vi "ProgramControl.vi"(0 "Universal Robot.lvclass in":refnum<class "Universal Robot.lvclass">, 1 "Program":string, 5 "error in (no error)":errorcluster, 8 "Timeout (s)":dbl=-1.0, 9 "Subpanel":refnum<vi>, 11 "Require Normal Mode to Play (F)":bool) -> (14 "Universal Robot.lvclass out":refnum<class "Universal Robot.lvclass">, 15 "programReturnStatus":T1=enum."Complete", 19 "error out":errorcluster)   [LabVIEW 2019, in "Universal Robot.lvclass"]
uses:
  Universal Robot.lvclass
  ProgramReturnStatus.ctl
  ProgramControlFPControls.ctl
  ProgramState.ctl
  Events/Robot Event/Event Type.ctl
  ProgramControlEvent.ctl
  Events/Robot Event/Robot Event.lvclass
panel:
  out "Loaded Program":string
  out "Program Status":string
  out "Program Status Color":u32(colorbox)
  out "Safety Status":string
  out "Safety Status Color":u32(colorbox)
  out "Time Elapsed":string
  out "Message":string
  in  "Abort":bool
  in  "Resume":bool
  in  "check status timeout":i32=1000
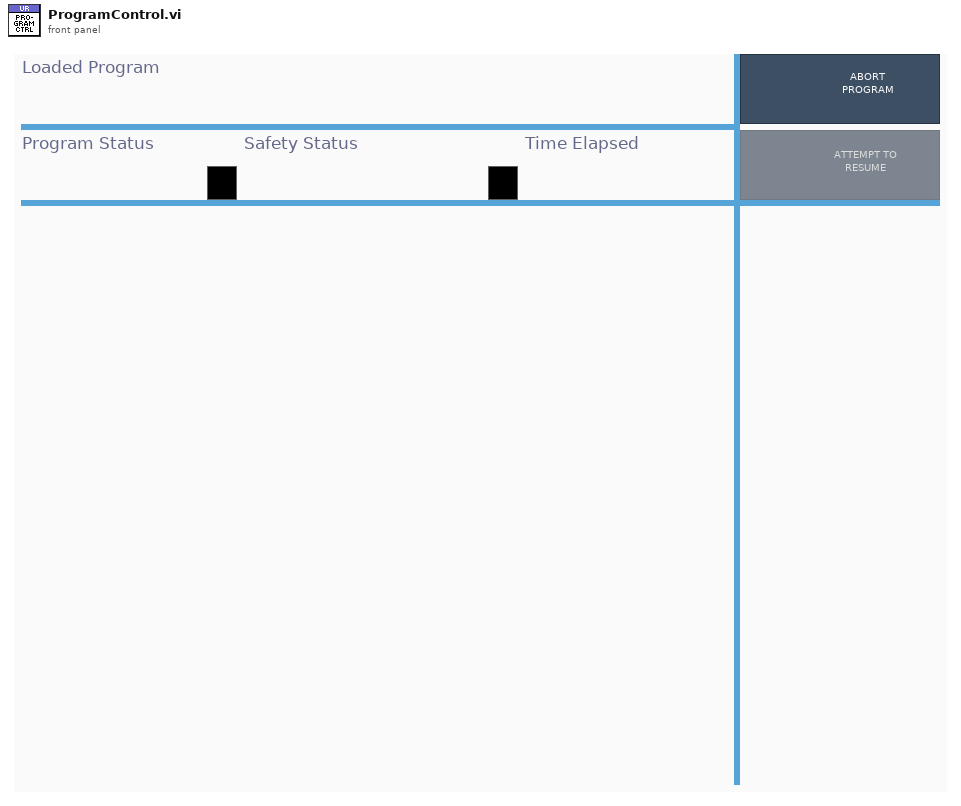
[diagram p1: front panel]
types:
  T1 = typedef "Universal Robot.lvclass/ProgramReturnStatus.ctl" = enum16{"Incomplete", "Complete", "Stopped", "User Stopped", "Error", "Faulted", "Timeout"}
  T2 = typedef "Universal Robot.lvclass/ProgramControlFPControls.ctl" = cluster{"Recover Button":refnum<vi>, "Resume Bottom":refnum<vi>, "Message":refnum<vi>, "Program Status":refnum<vi>, "Loaded Program":refnum<vi>, "VI Reference":refnum<vi>, "Time Elapsed":refnum<vi>, "Safety Status":refnum<vi>, "Program Status Color":refnum<vi>, "Safety Status Color":refnum<vi>}
  T3 = typedef "Universal Robot.lvclass/ProgramState.ctl" = enum16{"STOPPED", "PLAYING", "PAUSE"}
  T4 = typedef "Robot Event.lvclass/Event Type.ctl" = enum16{"Play", "Error", "Fault", "Timeout", "Stopped", "Complete", "Fault - Program Resumed", "Fault - Program Aborted"}
  T5 = typedef "Universal Robot.lvclass/ProgramControlEvent.ctl" = enum16{"Stop", "Pause", "Resume"}
  T6 = typedef "Universal Robot.lvclass/ProgramStatus.ctl" = cluster{"Loaded Program":string, "Valid Program":bool, "Program State":T3, "Running":bool}
  T7 = typedef "Universal Robot.lvclass/SafetyStatus.ctl" = enum16{"INVALID", "NORMAL", "REDUCED", "PROTECTIVE_STOP", "RECOVERY", "SAFEGUARD_STOP", "SYSTEM_EMERGENCY_STOP", "ROBOT_EMERGENCY_STOP", "VIOLATION", "FAULT", "AUTOMATIC_MODE_SAFEGAURD_STOP", "SYSTEM_THREE_POSITION_ENABLING_STOP"}
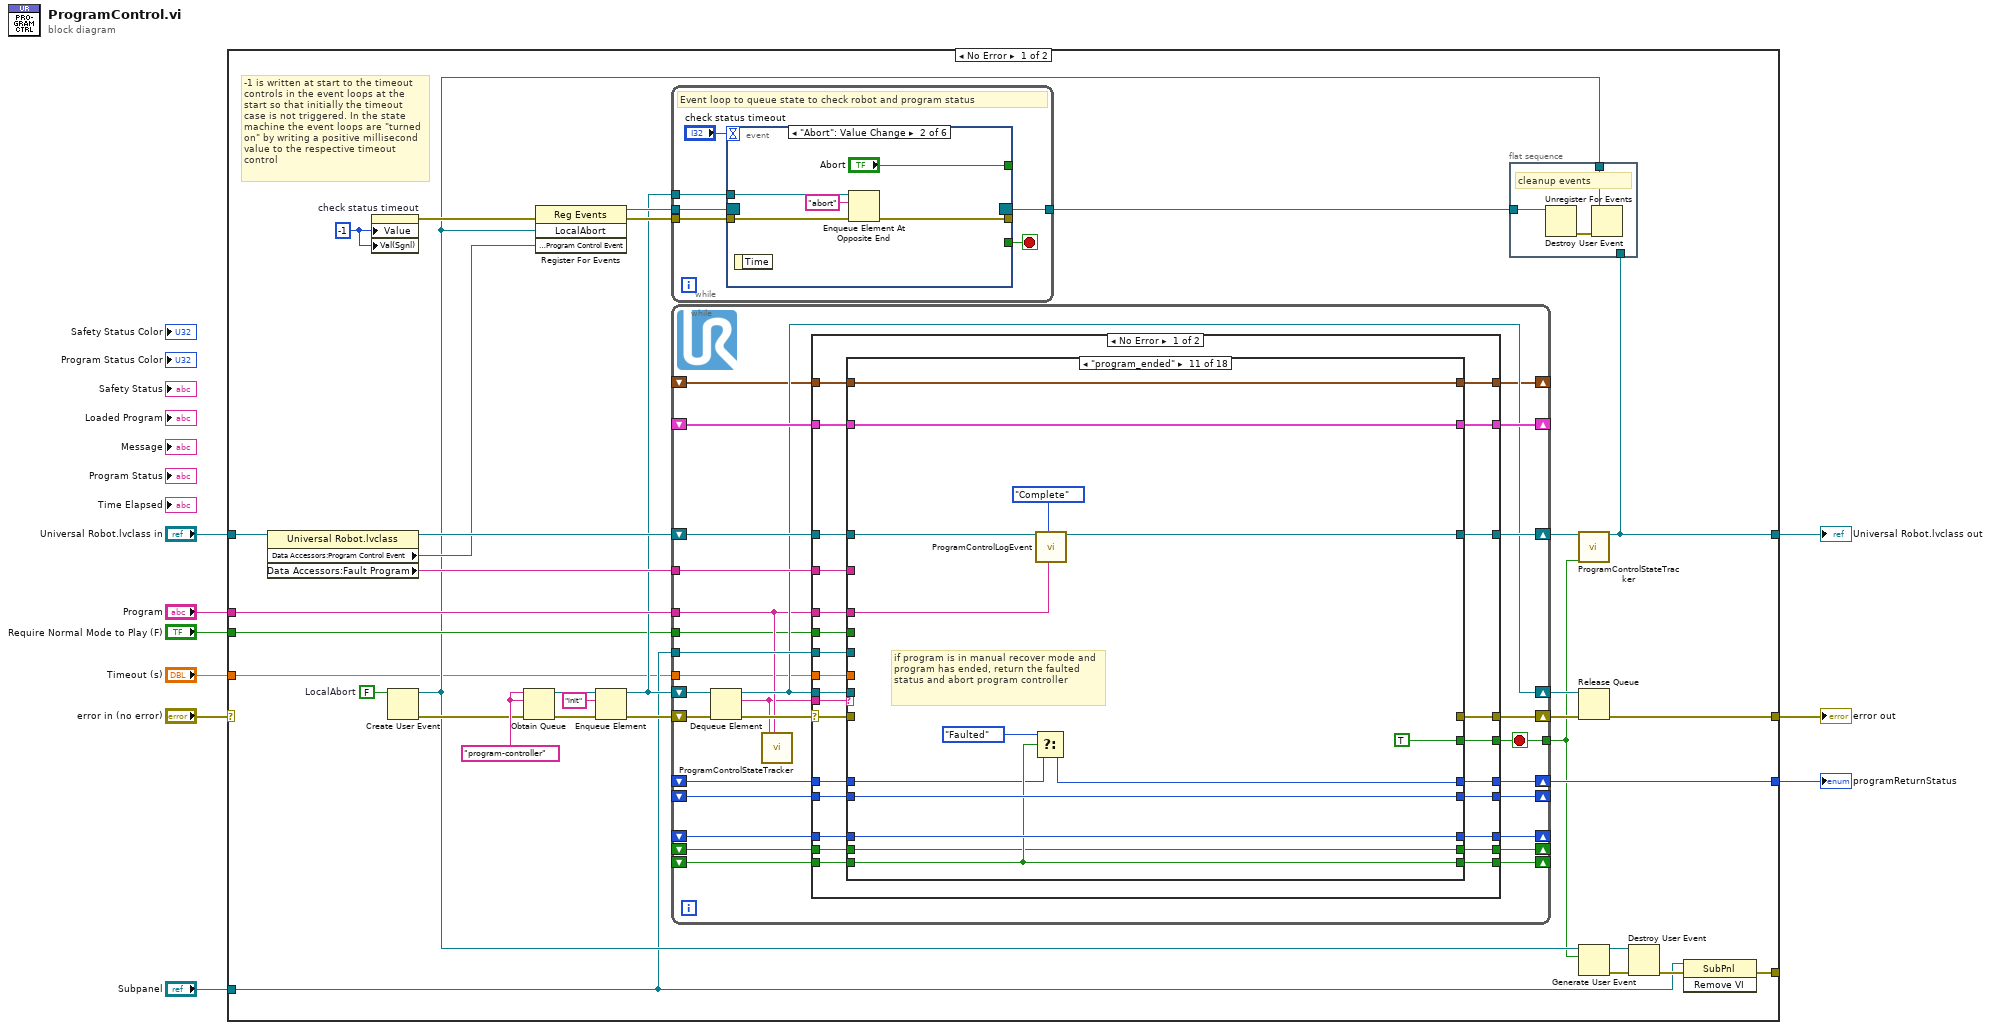
[diagram p0: block diagram]
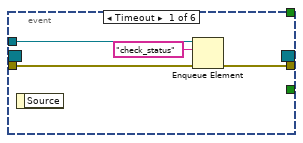
[diagram p2: hidden frame]
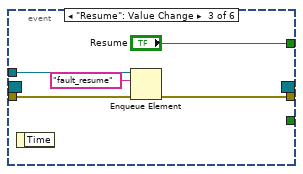
[diagram p3: hidden frame]
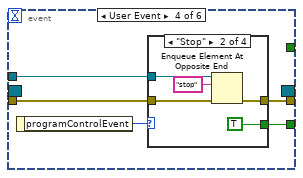
[diagram p4: hidden frame]
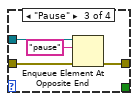
[diagram p6: hidden frame]
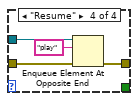
[diagram p7: hidden frame]
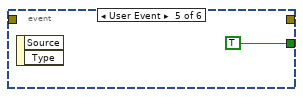
[diagram p8: hidden frame]
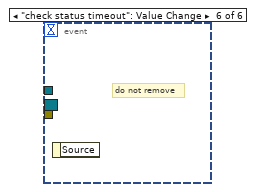
[diagram p9: hidden frame]
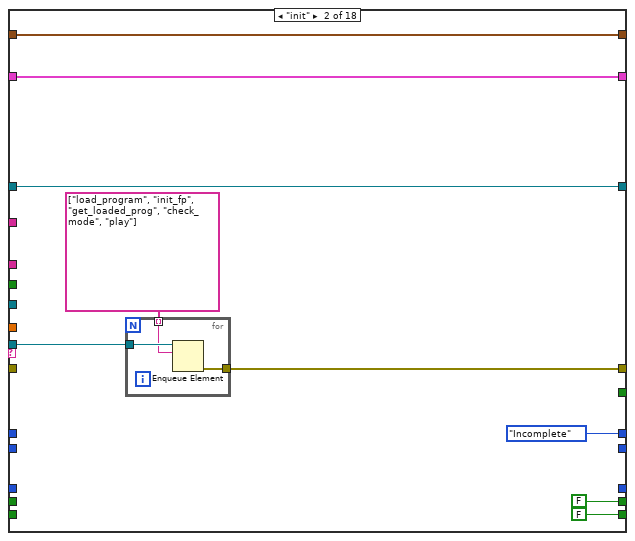
[diagram p11: hidden frame]
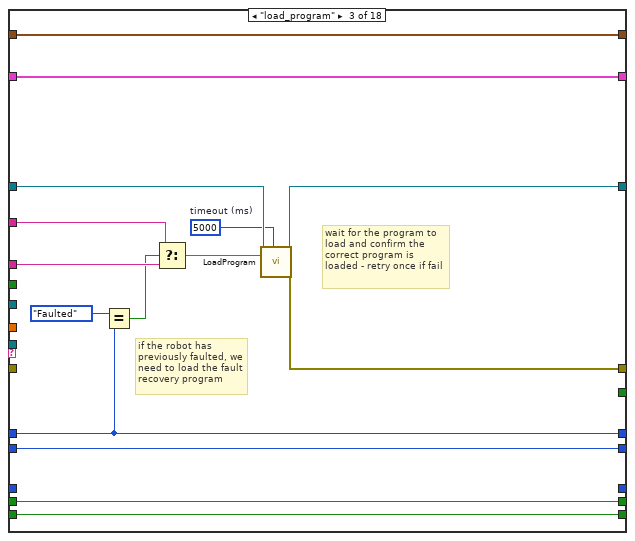
[diagram p12: hidden frame]
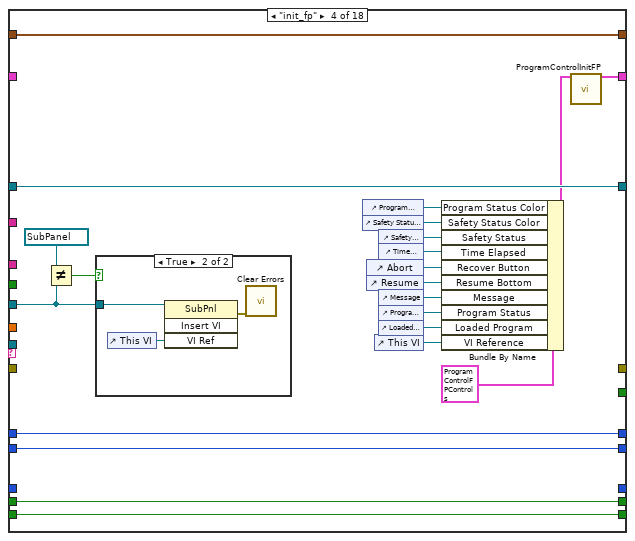
[diagram p13: hidden frame]
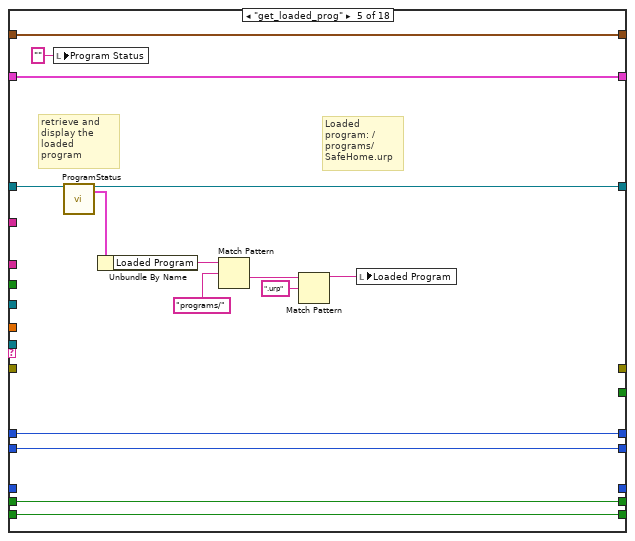
[diagram p15: hidden frame]
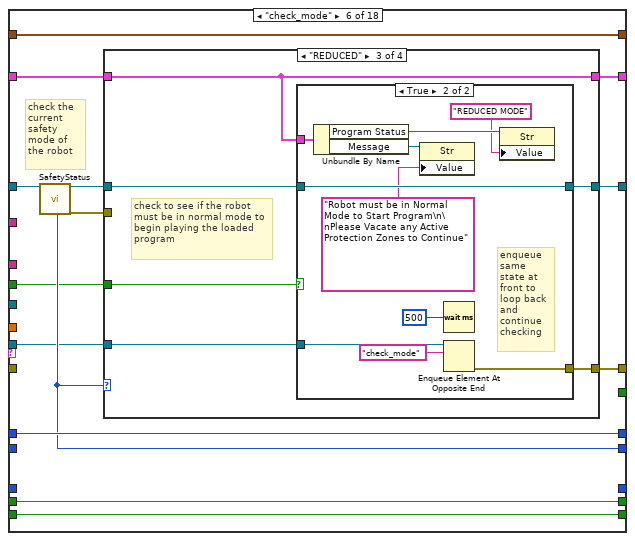
[diagram p16: hidden frame]
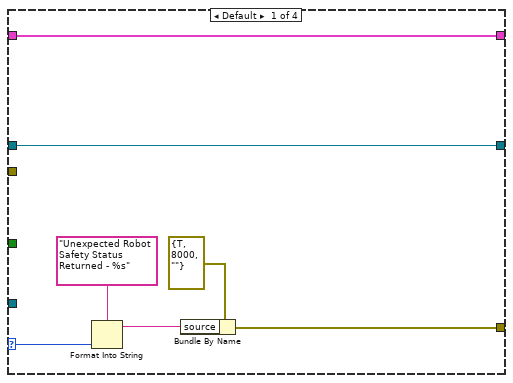
[diagram p17: hidden frame]
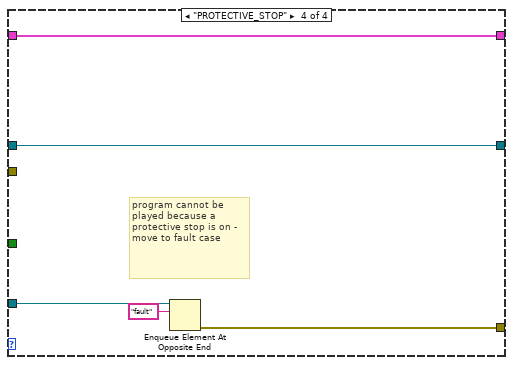
[diagram p20: hidden frame]
diagram:
  n1 = case shown="No Error" "error in (no error)" {
    selector: "error in (no error)" -> [_ w564]
    tunnel: "Universal Robot.lvclass in" -> [w33 w563]
    tunnel: [w31 _] -> w8
    tunnel: [w24 w564] -> w7
    tunnel: [w15 w563] -> w6
    tunnel: "Subpanel" -> [w12 _]
    tunnel: "Program" -> [w23 _]
    tunnel: "Require Normal Mode to Play (F)" -> [w18 _]
    tunnel: [w11 _] -> _
    tunnel: "Timeout (s)" -> [w10 _]
    frame No Error {
      w30 = FALSE  # LocalAbort
      w20 = -1 ("rate")
      w38 = "program-controller" ("name (unnamed)")
      # "-1 is written at start to the timeout controls in the event loops at the start so that initially the timeout case is not triggered. In the state machine the event loops are \"turned on\" by writing a positive millisecond value to the respective timeout control"
      n2 = property class="Universal Robot.lvclass"(reference=w33) -> (reference out=w37:refnum<class "Universal Robot.lvclass">, "Data Accessors:Program Control Event"=w32:refnum<user-event>, "Data Accessors:Fault Program"=w22:string)  [unwired: 1 in, 1 out]
      n3 = property on="check status timeout" class="DigNum (strict)"("Value"=w20, "Val(Sgnl)"=w20) -> (error out=w29:errorcluster)  [unwired: 2 in, 1 out]
      n4 = Create User Event(user event datatype=w30) -> (user event=w16:refnum<user-event>, error out=w28:errorcluster)  [unwired: 1 in]
      n5 = Obtain Queue(name (unnamed)=w38, element data type=w38, error in (no error)=w28) -> (queue out=w36:refnum<queue>, error out=w35:errorcluster)  [unwired: 2 in, 1 out]
      n6 = register-events(error in=w29, w16, w32) -> (reference out=w42:refnum<event-registration>, error out=w41:errorcluster)  [unwired: 1 in]
      n7 = Enqueue Element(queue=w36, element="init", error in (no error)=w35) -> (queue out=w21:refnum<queue>, error out=w34:errorcluster)  [unwired: 1 in, 1 out]
      n8 = while {
        tunnel: w21 -> [w51]
        tunnel: w41 -> [w50]
        tunnel: w42 -> [w49]
        tunnel: [w47] -> w17
        stop <- w46 stop-if-true
        # "Event loop to queue state to check robot and program status"
        n9 = event shown="[1] \"Abort\": Value Change" {
          selector: w49 -> [_ _ _ _ _ _]
          dyn-events: [_ _ _ _ _ _] -> w47
          timeout: "check status timeout" -> [_ _ _ _ _ _]
          tunnel: w51 -> [w55 w60 w65 w70 _ _]
          tunnel: w50 -> [w54 w59 w64 w69 _ _]
          tunnel: [w53 w58 w63 w68 _ _] -> _
          tunnel: [_ _ _ w66 TRUE _] -> w46
          tunnel: [_ "Abort" "Resume" _ _ _] -> _
          event Timeout {
            n10 = event-data() -> ()  [unwired: 1 in, 1 out]
            n11 = Enqueue Element(queue=w55, element="check_status", error in (no error)=w54) -> (error out=w53:errorcluster)  [unwired: 1 in, 2 out]
          }
          event "Abort": Value Change {
            n12 = event-data() -> ()  [unwired: 1 in, 1 out]
            n13 = Enqueue Element At Opposite End(queue=w60, element="abort", error in (no error)=w59) -> (error out=w58:errorcluster)  [unwired: 1 in, 2 out]
          }
          event "Resume": Value Change {
            n14 = event-data() -> ()  [unwired: 1 in, 1 out]
            n15 = Enqueue Element(queue=w65, element="fault_resume", error in (no error)=w64) -> (error out=w63:errorcluster)  [unwired: 1 in, 2 out]
          }
          event User Event {
            n16 = event-data() -> ("programControlEvent"=w67:T5)  [unwired: 1 in]
            n17 = case shown="\"Stop\"" w67 {
              tunnel: w70 -> [_ w76 w80 w84]
              tunnel: w69 -> [w71 w75 w79 w83]
              tunnel: [w71 w74 w78 w82] -> w68
              tunnel: [_ TRUE _ _] -> w66
              frame Default {
              }
              frame "Stop" {
                n18 = Enqueue Element At Opposite End(queue=w76, element="stop", error in (no error)=w75) -> (error out=w74:errorcluster)  [unwired: 1 in, 2 out]
              }
              frame "Pause" {
                n19 = Enqueue Element At Opposite End(queue=w80, element="pause", error in (no error)=w79) -> (error out=w78:errorcluster)  [unwired: 1 in, 2 out]
              }
              frame "Resume" {
                n20 = Enqueue Element At Opposite End(queue=w84, element="play", error in (no error)=w83) -> (error out=w82:errorcluster)  [unwired: 1 in, 2 out]
              }
            }
          }
          event User Event {
            n21 = event-data() -> ()  [unwired: 1 in, 2 out]
          }
          event "check status timeout": Value Change {
            # "do not remove"
            n22 = event-data() -> ()  [unwired: 1 in, 1 out]
          }
        }
      }
      n23 = while {
        shift-right: [w113] -> w40
        shift-left: w34 -> [w100]
        shift-right: [w99] -> w39
        shift-left: w21 -> [w101]
        shift-right: [w111] -> w19
        shift-left: w37 -> [w112]
        tunnel: [w109] -> w14
        tunnel: w12 -> [w108]
        shift-right: [w107] -> _
        shift-left: _ -> [w106]
        tunnel: w23 -> [w97]
        tunnel: w22 -> [w105]
        shift-right: [w110] -> w31
        shift-left: _ -> [w104]
        shift-right: [w103] -> _
        shift-left: _ -> [w102]
        tunnel: w18 -> [w96]
        shift-right: [w94] -> _
        shift-left: _ -> [w93]
        shift-right: [w92] -> _
        shift-left: _ -> [w91]
        tunnel: w10 -> [w90]
        shift-right: [w89] -> _
        shift-left: _ -> [w88]
        shift-right: [w87] -> _
        shift-left: _ -> [w86]
        stop <- w109 stop-if-true
        n24 = Dequeue Element(queue=w101, error in (no error)=w100) -> (queue out=w99:refnum<queue>, element=w95:string, error out=w98:errorcluster)  [unwired: 1 in, 1 out]
        n25 = call "ProgramControlStateTracker.vi"("State in"=w95, "Program"=w97) -> ()  [unwired: 17 in, 1 out]
        n26 = case shown="No Error" w98 {
          selector: w98 -> [w125 w557]
          tunnel: w99 -> [w126 _]
          tunnel: [w139 w557] -> w113
          tunnel: [w138 TRUE] -> w109
          tunnel: w112 -> [w137 w554]
          tunnel: [w136 w552] -> w111
          tunnel: [w135 ProgramReturnStatus."Error" ("programReturnStatus")] -> w110
          tunnel: w108 -> [w134 _]
          tunnel: [w133 w560] -> w107
          tunnel: w106 -> [w132 w560]
          tunnel: w97 -> [w129 w551]
          tunnel: w105 -> [w131 _]
          tunnel: w104 -> [w130 _]
          tunnel: [w128 w559] -> w103
          tunnel: w102 -> [w127 w559]
          tunnel: w95 -> [w124 _]
          tunnel: w96 -> [w123 _]
          tunnel: [w122 w549] -> w94
          tunnel: w93 -> [w121 w549]
          tunnel: [w120 w550] -> w92
          tunnel: w91 -> [w119 w550]
          tunnel: w90 -> [w118 _]
          tunnel: [w117 w548] -> w89
          tunnel: w88 -> [w116 w548]
          tunnel: [w115 w547] -> w87
          tunnel: w86 -> [w114 w547]
          frame No Error {
            n27 = case shown="\"program_ended\"" w124 {
              tunnel: w125 -> [w147 _ _ _ _ _ _ _ _ _ _ w405 w428 _ w459 _ _ _]
              tunnel: w126 -> [_ w154 _ _ _ w225 w275 _ _ w331 _ w412 w434 w444 w475 w492 _ _]
              tunnel: [w147 w153 w160 _ _ w226 w276 errorcluster {"status"=TRUE, "code"=8000, "source"="Timed out waiting for program to play"} ("error out") _ w330 _ w401 w418 w443 w464 w487 w531 w542] -> w139
              tunnel: [_ _ _ _ _ _ _ TRUE _ _ TRUE _ _ _ _ w480 TRUE _] -> w138
              tunnel: w137 -> [w146 w156 w173 w187 w214 w223 w280 w302 w310 w323 w387 w410 w433 w442 w468 w489 w532 w546]
              tunnel: [w146 w156 w161 w187 w213 w221 w268 w302 w310 w329 w385 w409 w432 w441 w466 w491 w517 w543] -> w136
              tunnel: [w144 ProgramReturnStatus."Incomplete" ("programReturnStatus") w169 w188 w206 w228 w270 ProgramReturnStatus."Error" ("programReturnStatus") w307 w325 w390 w411 ProgramReturnStatus."Timeout" ("programReturnStatus") w437 w471 ProgramReturnStatus."Faulted" ("programReturnStatus") w520 w538] -> w135
              tunnel: w134 -> [_ _ _ w196 _ _ _ _ _ _ _ _ _ _ _ _ _ _]
              tunnel: [w145 w155 w174 w189 w205 w218 w263 w299 w308 w328 w397 w413 w423 w447 w472 w494 w528 w540] -> w133
              tunnel: w132 -> [w145 w155 w174 _ w205 w219 w263 w299 w308 w320 w397 w414 w423 w447 w473 w494 w528 w540]
              tunnel: w129 -> [_ _ w172 _ _ _ w266 _ _ _ w386 w408 w431 _ w465 w488 w515 _]
              tunnel: w131 -> [_ _ w171 _ _ _ _ _ _ _ _ _ _ _ _ w483 _ _]
              tunnel: w130 -> [w144 _ w169 w188 w206 w228 w270 _ w307 w326 w392 w411 _ w439 w471 _ w521 w538]
              tunnel: [w143 _ w166 w184 w204 w227 w265 w297 w306 w327 w395 w406 w429 w436 w470 w490 w527 w537] -> w128
              tunnel: w127 -> [w143 _ w166 w184 w204 _ w265 w297 w306 w324 w395 w406 w429 w438 w470 w490 w527 w537]
              tunnel: w123 -> [_ _ _ _ _ w220 _ _ _ _ _ _ _ _ _ _ _ _]
              tunnel: [_ _ _ _ _ _ _ _ _ w319 w394 w403 w426 _ _ _ _ _] -> w122
              tunnel: w121 -> [_ _ _ _ _ _ _ _ _ _ w394 w403 w426 _ _ _ _ _]
              tunnel: [w142 FALSE w165 w181 w202 w217 w262 w296 w305 w318 w393 w400 w425 w446 w462 TRUE w526 w536] -> w120
              tunnel: w119 -> [w142 _ w165 w181 w202 w217 w262 w296 w305 w318 w393 w400 w425 w446 w462 w482 w526 w536]
              tunnel: w118 -> [_ _ _ _ _ _ _ _ _ w317 _ _ w422 _ _ _ _ _]
              tunnel: [w141 w149 w164 w180 w201 w216 w261 w295 w304 w315 w389 w399 w424 w445 w461 w486 w525 w535] -> w117
              tunnel: w116 -> [w141 w149 w164 w180 w201 w216 w261 w295 _ w315 w389 w399 w424 w445 w461 w486 w525 w535]
              tunnel: [w140 FALSE w163 w175 w200 w215 FALSE w294 w303 w311 w388 TRUE w416 w440 w460 w479 w519 w534] -> w115
              tunnel: w114 -> [w140 _ w163 w175 w200 w215 _ w294 w303 w311 w388 _ w416 w440 w460 w479 w519 w534]
              frame Default {
              }
              frame "init" {
                n28 = for {
                  tunnel: w154 -> [w159]
                  tunnel: [w158] -> w153
                  tunnel: string[] ["load_program", "init_fp", "get_loaded_prog", "check_mode", "play"] -> [w157] mode=indexing
                  n29 = Enqueue Element(queue=w159, element=w157) -> (error out=w158:errorcluster)  [unwired: 2 in, 2 out]
                }
              }
              frame "load_program" {
                w162 = u32 5000  # timeout (ms)
                # "wait for the program to load and confirm the correct program is loaded - retry once if fail"
                # "if the robot has previously faulted, we need to load the fault recovery program"
                n30 = Equal?(x=ProgramReturnStatus."Faulted", y=w169) -> (x = y?=w167:bool)
                n31 = Select(t=w171, s=w167, f=w172) -> (s? t:f=w170:string)
                n32 = call-dynamic "LoadProgram.vi"("Universal Robot.lvclass in"=w173, "program in"=w170, "timeout (ms)"=w162) -> ("Universal Robot.lvclass out"=w161:refnum<class "Universal Robot.lvclass">, "error out"=w160:errorcluster)  [unwired: 14 in, 1 out]
              }
              frame "init_fp" {
                n33 = Not Equal?(x=refnum<vi> refnum, y=w196) -> (x != y?=w194:bool)
                n34 = case shown="True" w194 {
                  tunnel: w196 -> [_ w199]
                  frame False {
                  }
                  frame True {
                    n35 = control-ref of="This VI"() -> (w197:refnum<vi>)
                    n36 = invoke class="SubPnl" method="Insert VI"(reference=w199, "VI Ref"=w197) -> (error out=w198:errorcluster)  [unwired: 2 in, 3 out]
                    n37 = call <vilib>:"Clear Errors.vi"("error in (no error)"=w198) -> ()  [unwired: 5 in, 2 out]
                  }
                }
                n38 = control-ref of="Program Status Color"() -> (w177:refnum<vi>)
                n39 = control-ref of="Safety Status Color"() -> (w176:refnum<vi>)
                n40 = control-ref of="Abort"() -> (w193:refnum<vi>)
                n41 = control-ref of="Resume"() -> (w192:refnum<vi>)
                n42 = control-ref of="This VI"() -> (w182:refnum<vi>)
                n43 = control-ref of="Safety Status"() -> (w178:refnum<vi>)
                n44 = control-ref of="Time Elapsed"() -> (w179:refnum<vi>)
                n45 = control-ref of="Message"() -> (w191:refnum<vi>)
                n46 = control-ref of="Program Status"() -> (w190:refnum<vi>)
                n47 = control-ref of="Loaded Program"() -> (w183:refnum<vi>)
                n48 = Bundle By Name(cluster=T2 {"Recover Button"=refnum, "Resume Bottom"=refnum, "Message"=refnum, "Program Status"=refnum, "Loaded Program"=refnum, "VI Reference"=refnum, "Time Elapsed"=refnum, "Safety Status"=refnum, "Program Status Color"=refnum, "Safety Status Color"=refnum} ("Front Panel Controls"), "Program Status Color"=w177, "Safety Status Color"=w176, "Safety Status"=w178, "Time Elapsed"=w179, "Recover Button"=w193, "Resume Bottom"=w192, "Message"=w191, "Program Status"=w190, "Loaded Program"=w183, "VI Reference"=w182) -> (w185:T2)
                n49 = call "ProgramControlInitFP.vi"("Front Panel Controls in"=w185) -> ("Front Panel Controls out"=w189:T2)  [unwired: 18 in]
              }
              frame "get_loaded_prog" {
                # "Loaded program: /programs/SafeHome.urp"
                # "retrieve and display the loaded program"
                n50 = local write "Program Status"("" ("Program Status")) -> ()
                n51 = call-dynamic "ProgramStatus.vi"("Universal Robot.lvclass in"=w214) -> ("Universal Robot.lvclass out"=w213:refnum<class "Universal Robot.lvclass">, "Program Status"=w212:T6)  [unwired: 16 in, 1 out]
                n52 = Unbundle By Name(w212) -> ("Loaded Program"=w210:string)
                n53 = Match Pattern(string=w210, regular expression="programs/") -> (after substring=w208:string)  [unwired: 1 in, 3 out]
                n54 = Match Pattern(string=w208, regular expression=".urp") -> (before substring=w203:string)  [unwired: 1 in, 3 out]
                n55 = local write "Loaded Program"(w203) -> ()
              }
              frame "check_mode" {
                # "check the current safety mode of the robot"
                n56 = call-dynamic "SafetyStatus.vi"("Universal Robot.lvclass in"=w223) -> ("safetyStatus out"=w227:T7, "Universal Robot.lvclass out"=w222:refnum<class "Universal Robot.lvclass">, "error out"=w224:errorcluster)  [unwired: 16 in]
                n57 = case shown="\"REDUCED\"" w227 {
                  selector: w227 -> [w231 _ _ _]
                  tunnel: w224 -> [_ _ _ _]
                  tunnel: [w232 _ w242 w258] -> w226
                  tunnel: w225 -> [_ _ w243 w259]
                  tunnel: w222 -> [w230 w237 w240 w256]
                  tunnel: [w230 w237 w241 w256] -> w221
                  tunnel: w220 -> [_ _ w239 _]
                  tunnel: w219 -> [w229 w236 w238 w255]
                  tunnel: [w229 w236 w238 w255] -> w218
                  frame Default {
                    n58 = Format Into String(format string="Unexpected Robot Safety Status Returned - %s", w231) -> (resulting string=w235:string)  [unwired: 2 in, 1 out]
                    n59 = Bundle By Name(cluster=errorcluster {"status"=TRUE, "code"=8000, "source"=""} ("error constant"), "source"=w235) -> (w232:errorcluster)
                  }
                  frame "NORMAL" {
                  }
                  frame "REDUCED" {
                    # "check to see if the robot must be in normal mode to begin playing the loaded program"
                    n60 = case shown="True" w239 {
                      tunnel: w243 -> [_ w254]
                      tunnel: [_ w253] -> w242
                      tunnel: w240 -> [w244 w249]
                      tunnel: [w244 w249] -> w241
                      tunnel: w238 -> [_ w247]
                      frame False {
                      }
                      frame True {
                        # "enqueue same state at front to loop back and continue checking"
                        n61 = Unbundle By Name(w247) -> ("Program Status"=w246:refnum<vi>, "Message"=w250:refnum<vi>)
                        n62 = property class="Str"(reference=w250, "Value"="Robot must be in Normal Mode to Start Program\n\nPlease Vacate any Active Protection Zones to Continue" ("element")) -> ()  [unwired: 1 in, 2 out]
                        n63 = Wait (ms)(milliseconds to wait=u32 500) -> ()  [unwired: 1 out]
                        n64 = Enqueue Element At Opposite End(queue=w254, element="check_mode") -> (error out=w253:errorcluster)  [unwired: 2 in, 2 out]
                        n65 = property class="Str"(reference=w246, "Value"="REDUCED MODE" ("element")) -> ()  [unwired: 1 in, 2 out]
                      }
                    }
                  }
                  frame "PROTECTIVE_STOP" {
                    # "program cannot be played because a protective stop is on - move to fault case"
                    n66 = Enqueue Element At Opposite End(queue=w259, element="fault") -> (error out=w258:errorcluster)  [unwired: 2 in, 2 out]
                  }
                }
              }
              frame "play" {
                # "play the program and wait  until it begins playing or a timeout is reached"
                n67 = call-dynamic "Play.vi"("Universal Robot.lvclass in"=w280) -> ("Universal Robot.lvclass out"=w279:refnum<class "Universal Robot.lvclass">, "error out"=w278:errorcluster)  [unwired: 17 in]
                n68 = Tick Count (ms)() -> (millisecond timer value=w277:u32)
                n69 = while {
                  shift-right: [w282] -> w269
                  shift-left: w279 -> [w285]
                  tunnel: w278 -> [w284]
                  tunnel: w277 -> [w292]
                  tunnel: [w283] -> w264
                  tunnel: [w290] -> w274
                  tunnel: [w286] -> w267
                  stop <- w287 stop-if-true
                  # "Wait for program to start"
                  n70 = call-dynamic "ProgramState.vi"("Universal Robot.lvclass in"=w285, "error in (no error)"=w284) -> ("Universal Robot.lvclass out"=w282:refnum<class "Universal Robot.lvclass">, "programState out"=w281:T3, "error out"=w283:errorcluster)  [unwired: 15 in]
                  n71 = Tick Count (ms)() -> (millisecond timer value=w293:u32)
                  n72 = Subtract(x=w293, y=w292) -> (x-y=w286:u32)
                  n73 = Greater?(x=w286, y=u32 5000) -> (0:w290:bool)
                  n74 = Equal?(x=ProgramState."PLAYING", y=w281) -> (x = y?=w288:bool)
                  n75 = Or(x=w288, y=w290) -> (x .or. y?=w287:bool)
                }
                n76 = Select(t="startup_error", s=w274, f="start_program_control") -> (s? t:f=w272:string)
                n77 = Enqueue Element(queue=w275, element=w272, error in (no error)=w264) -> (error out=w276:errorcluster)  [unwired: 1 in, 2 out]
                n78 = call "ProgramControlLogEvent.vi"("Universal Robot.lvclass"=w269, "data"=w267, "Program"=w266) -> ("Universal Robot.lvclass out"=w268:refnum<class "Universal Robot.lvclass">)  [unwired: 16 in]
              }
              frame "startup_error" {
                # "the application timed out waiting for the loaded program to start\n\ncheck the teach pendant for errors"
              }
              frame "start_program_control" {
                w309 = 500 ("rate")
                # "turn on timeout event which is used to check program status"
                n79 = property on="check status timeout" class="DigNum (strict)"("Value"=w309, "Val(Sgnl)"=w309) -> ()  [unwired: 2 in, 2 out]
                n80 = Get Date/Time In Seconds() -> (seconds since 1Jan1904=w304:timestamp)
              }
              frame "check_status" {
                # "get time elapsed"
                # "check the robot safety status"
                n81 = call-dynamic "SafetyStatus.vi"("Universal Robot.lvclass in"=w323) -> ("safetyStatus out"=w319:T7, "Universal Robot.lvclass out"=w322:refnum<class "Universal Robot.lvclass">, "error out"=w321:errorcluster)  [unwired: 16 in]
                n82 = Get Date/Time In Seconds() -> (seconds since 1Jan1904=w316:timestamp)
                n83 = call "ProgramControlSafetyMode.vi"("Front Panel Controls in"=w320, "Safety Status"=w319) -> ("Front Panel Controls out"=w314:T2)  [unwired: 17 in]
                n84 = Subtract(x=w316, y=w315) -> (x-y=w312:dbl)
                n85 = call "ProgramControlTiming.vi"("Front Panel Controls in"=w314, "Time Elapsed"=w312) -> ("Front Panel Controls out"=w313:T2)  [unwired: 17 in]
                n86 = case shown="\"NORMAL\", \"REDUCED\"" w319 {
                  selector: w319 -> [w343 _ w378]
                  tunnel: w331 -> [w345 w371 _]
                  tunnel: [w344 w372 w376] -> w330
                  tunnel: [w339 w374 w383] -> w329
                  tunnel: w322 -> [w342 w374 w383]
                  tunnel: w321 -> [w341 _ _]
                  tunnel: w313 -> [w334 w370 w382]
                  tunnel: [w333 w370 w382] -> w328
                  tunnel: [w343 w369 w381] -> w327
                  tunnel: w326 -> [w338 w368 w380]
                  tunnel: [w337 w368 w380] -> w325
                  tunnel: w324 -> [_ w369 w381]
                  tunnel: w317 -> [w336 _ _]
                  tunnel: w312 -> [w335 _ _]
                  frame "NORMAL", "REDUCED" {
                    # "determine if the program has completed or timed out if a timeout value is defined"
                    n87 = call-dynamic "ProgramState.vi"("Universal Robot.lvclass in"=w342, "error in (no error)"=w341) -> ("Universal Robot.lvclass out"=w339:refnum<class "Universal Robot.lvclass">, "programState out"=w332:T3, "error out"=w340:errorcluster)  [unwired: 15 in]
                    n88 = case shown="\"STOPPED\"" w332 {
                      tunnel: w345 -> [w354 w359]
                      tunnel: w340 -> [w353 _]
                      tunnel: [w352 w360] -> w344
                      tunnel: w338 -> [w347 w361]
                      tunnel: [w348 w361] -> w337
                      tunnel: w336 -> [_ w358]
                      tunnel: w335 -> [_ w356]
                      frame "STOPPED" {
                        w346 = ProgramReturnStatus."User Stopped" ("x")
                        # "determine if program stopped because it was completed or if it was aborted by user"
                        n89 = Not Equal?(x=w347, y=w346) -> (x != y?=w350:bool)
                        n90 = Enqueue Element At Opposite End(queue=w354, element="program_ended", error in (no error)=w353) -> (error out=w352:errorcluster)  [unwired: 1 in, 2 out]
                        n91 = Select(t=ProgramReturnStatus."Complete" ("programReturnStatus"), s=w350, f=w346) -> (s? t:f=w348:T1)
                      }
                      frame Default {
                        n92 = Greater Than 0?(x=w358) -> (x > 0?=w357:bool)
                        n93 = Greater?(x=w356, y=w358) -> (0:w355:bool)
                        n94 = case shown="True" w357 {
                          tunnel: [_ w364] -> w360
                          tunnel: w359 -> [_ w363]
                          tunnel: w355 -> [_ w362]
                          frame False {
                            # "no timeout value defined"
                          }
                          frame True {
                            n95 = case shown="True" w362 {
                              tunnel: [_ w367] -> w364
                              tunnel: w363 -> [_ w366]
                              frame False {
                              }
                              frame True {
                                n96 = Enqueue Element At Opposite End(queue=w366, element="timeout") -> (error out=w367:errorcluster)  [unwired: 2 in, 2 out]
                              }
                            }
                          }
                        }
                      }
                    }
                    n97 = call "ProgramControlProgramStatus.vi"("Front Panel Controls in"=w334, "Program State"=w332) -> ("Front Panel Controls out"=w333:T2)  [unwired: 17 in]
                  }
                  frame "PROTECTIVE_STOP" {
                    # "protective stop was triggered, alert the user"
                    n98 = Enqueue Element At Opposite End(queue=w371, element="fault") -> (error out=w372:errorcluster)  [unwired: 2 in, 2 out]
                  }
                  frame Default {
                    # "an unhandled safety status was returned, need to create an error"
                    n99 = Format Into String(format string="Unexpected Robot Safety Status Returned - %s", w378) -> (resulting string=w375:string)  [unwired: 2 in, 1 out]
                    n100 = Bundle By Name(cluster=errorcluster {"status"=TRUE, "code"=8000, "source"=""} ("error constant"), "source"=w375) -> (w376:errorcluster)
                  }
                }
              }
              frame "program_ended" {
                # "if program is in manual recover mode and program has ended, return the faulted status and abort program controller"
                n101 = Select(t=ProgramReturnStatus."Faulted" ("programReturnStatus"), s=w393, f=w392) -> (s? t:f=w390:T1)
                n102 = call "ProgramControlLogEvent.vi"("Universal Robot.lvclass"=w387, "Event Type"=Event_Type."Complete", "Program"=w386) -> ("Universal Robot.lvclass out"=w385:refnum<class "Universal Robot.lvclass">)  [unwired: 16 in]
              }
              frame "fault" {
                w415 = -1 ("rate")
                # "set flag that program has faulted"
                # "flush queue to prevent strange behavior"
                # "check status event loop is temporarily disabled"
                # "make fault recovery buttons visible"
                n103 = Format Into String(w403) -> (resulting string=w402:string)  [unwired: 3 in, 1 out]
                n104 = property on="check status timeout" class="DigNum (strict)"(error in=w405, "Value"=w415, "Val(Sgnl)"=w415) -> (error out=w404:errorcluster)  [unwired: 1 in, 1 out]
                n105 = call "ProgramControlFault.vi"("Front Panel Controls in"=w414) -> ("Front Panel Controls out"=w413:T2)  [unwired: 18 in]
                n106 = call "ProgramControlLogEvent.vi"("Universal Robot.lvclass"=w410, "data"=w402, "Event Type"=Event_Type."Fault", "Program"=w408) -> ("Universal Robot.lvclass out"=w409:refnum<class "Universal Robot.lvclass">)  [unwired: 15 in]
                n107 = Flush Queue(queue=w412, error in (no error)=w404) -> (error out=w401:errorcluster)  [unwired: 2 out]
              }
              frame "timeout" {
                w435 = -1 ("rate")
                # "flush queue to prevent strange behavior"
                # "check status event loop is temporarily disabled"
                n108 = property on="check status timeout" class="DigNum (strict)"(error in=w428, "Value"=w435, "Val(Sgnl)"=w435) -> (error out=w427:errorcluster)  [unwired: 1 in, 1 out]
                n109 = call "ProgramControlLogEvent.vi"("Universal Robot.lvclass"=w433, "data"=w422, "Event Type"=Event_Type."Timeout", "Program"=w431) -> ("Universal Robot.lvclass out"=w432:refnum<class "Universal Robot.lvclass">)  [unwired: 15 in]
                n110 = Flush Queue(queue=w434, error in (no error)=w427) -> (queue out=w420:refnum<queue>, error out=w419:errorcluster)  [unwired: 1 out]
                n111 = Enqueue Element(queue=w420, element="stop", error in (no error)=w419) -> (error out=w418:errorcluster)  [unwired: 1 in, 2 out]
              }
              frame "abort" {
                n112 = case shown="False" w440 {
                  tunnel: w444 -> [w453 _]
                  tunnel: [w452 _] -> w443
                  tunnel: w442 -> [w450 w458]
                  tunnel: [w450 w457] -> w441
                  tunnel: w439 -> [w449 _]
                  tunnel: w438 -> [w448 w455]
                  tunnel: [w449 ProgramReturnStatus."User Stopped" ("programReturnStatus")] -> w437
                  tunnel: [w448 w455] -> w436
                  frame True {
                    n113 = Enqueue Element At Opposite End(queue=w453, element="fault_abort") -> (error out=w452:errorcluster)  [unwired: 2 in, 2 out]
                  }
                  frame False {
                    n114 = call-dynamic "ProgramRemote.vi"("Universal Robot.lvclass in"=w458, "Remote"=ProgramControlEvent."Stop") -> ("Universal Robot.lvclass out"=w457:refnum<class "Universal Robot.lvclass">)  [unwired: 16 in, 1 out]
                  }
                }
              }
              frame "fault_resume" {
                # "unlock the protective stop and attempt to recover the fault by sending play to resume the loaded program from the current execution spot"
                n115 = call "ProgramControlLogEvent.vi"("Universal Robot.lvclass"=w468, "Event Type"=Event_Type."Fault - Program Resumed", "Program"=w465) -> ("Universal Robot.lvclass out"=w467:refnum<class "Universal Robot.lvclass">)  [unwired: 16 in]
                n116 = call-dynamic "UnlockProtectiveStop.vi"("Universal Robot.lvclass in"=w467, "error in (no error)"=w459) -> ("Universal Robot.lvclass out"=w466:refnum<class "Universal Robot.lvclass">, "error out"=w463:errorcluster)  [unwired: 16 in]
                n117 = case shown="No Error" w463 {
                  tunnel: w473 -> [w477 w478]
                  tunnel: [w476 w478] -> w472
                  frame No Error {
                    n118 = call "ProgramControlInitFP.vi"("Front Panel Controls in"=w477) -> ("Front Panel Controls out"=w476:T2)  [unwired: 18 in]
                  }
                  frame Error {
                  }
                }
                n119 = Enqueue Element(queue=w475, element="play", error in (no error)=w463) -> (error out=w464:errorcluster)  [unwired: 1 in, 2 out]
              }
              frame "fault_abort" {
                n120 = call "ProgramControlLogEvent.vi"("Universal Robot.lvclass"=w489, "Event Type"=Event_Type."Fault - Program Aborted", "Program"=w488) -> ("Universal Robot.lvclass out"=w485:refnum<class "Universal Robot.lvclass">)  [unwired: 16 in]
                n121 = case shown="Default" w483 {
                  tunnel: w492 -> [_ w502]
                  tunnel: [w496 w501] -> w491
                  tunnel: [_ w500] -> w487
                  tunnel: w485 -> [w496 w499]
                  tunnel: w482 -> [_ w498]
                  tunnel: [TRUE w497] -> w480
                  frame "" {
                    # "there is no fault program defined so close the program controller"
                  }
                  frame Default {
                    # "a fault program is defined which is run on abort condition"
                    n122 = case shown="False" w498 {
                      tunnel: w502 -> [w508 _]
                      tunnel: [w507 w514] -> w501
                      tunnel: [w506 _] -> w500
                      tunnel: w499 -> [w503 w514]
                      tunnel: [_ TRUE] -> w497
                      frame False {
                        n123 = call-dynamic "UnlockProtectiveStop.vi"("Universal Robot.lvclass in"=w503) -> ("Universal Robot.lvclass out"=w507:refnum<class "Universal Robot.lvclass">, "error out"=w504:errorcluster)  [unwired: 17 in]
                        n124 = for {
                          tunnel: w508 -> [w512]
                          tunnel: [w511] -> w506
                          tunnel: string[] ["load_program", "get_loaded_prog", "play"] -> [w510] mode=indexing
                          tunnel: w504 -> [w509]
                          n125 = Enqueue Element(queue=w512, element=w510, error in (no error)=w509) -> (error out=w511:errorcluster)  [unwired: 1 in, 2 out]
                        }
                      }
                      frame True {
                        # "already attempted to run the fault program, abort the program controller"
                      }
                    }
                  }
                }
              }
              frame "stop" {
                w530 = -1 ("rate")
                # "check to see if the program stopped because of a timeout or because it was finished"
                n126 = property on="check status timeout" class="DigNum (strict)"("Value"=w530, "Val(Sgnl)"=w530) -> (error out=w529:errorcluster)  [unwired: 2 in, 1 out]
                n127 = Not Equal?(x=ProgramReturnStatus."Timeout", y=w521) -> (x != y?=w523:bool)
                n128 = Select(t=ProgramReturnStatus."Stopped" ("programReturnStatus"), s=w523, f=w521) -> (s? t:f=w520:T1)
                n129 = call-dynamic "Stop.vi"("Universal Robot.lvclass in"=w532, "error in (no error)"=w529) -> ("Universal Robot.lvclass out"=w518:refnum<class "Universal Robot.lvclass">, "error out"=w531:errorcluster)  [unwired: 16 in]
                n130 = call "ProgramControlLogEvent.vi"("Universal Robot.lvclass"=w518, "Event Type"=Event_Type."Stopped", "Program"=w515) -> ("Universal Robot.lvclass out"=w517:refnum<class "Universal Robot.lvclass">)  [unwired: 16 in]
              }
              frame "pause" {
                w545 = -1 ("rate")
                n131 = property on="check status timeout" class="DigNum (strict)"("Value"=w545, "Val(Sgnl)"=w545) -> (error out=w544:errorcluster)  [unwired: 2 in, 1 out]
                n132 = Unbundle By Name(w540) -> ("Program Status"=w541:refnum<vi>)
                n133 = call-dynamic "Pause.vi"("Universal Robot.lvclass in"=w546, "error in (no error)"=w544) -> ("Universal Robot.lvclass out"=w543:refnum<class "Universal Robot.lvclass">, "error out"=w542:errorcluster)  [unwired: 16 in]
                n134 = property class="Str"(reference=w541, "Value"="PAUSED") -> ()  [unwired: 1 in, 2 out]
              }
            }
          }
          frame Error {
            n135 = Unbundle By Name(w557) -> ("source"=w556:string)
            n136 = call "ProgramControlLogEvent.vi"("Universal Robot.lvclass"=w554, "data"=w556, "Event Type"=Event_Type."Error", "Program"=w551) -> ("Universal Robot.lvclass out"=w553:refnum<class "Universal Robot.lvclass">)  [unwired: 15 in]
            n137 = call "ProgramControlStateTracker.vi"("Universal Robot.lvclass"=w553, "State in"="error", "Program"=w551) -> ("Universal Robot.lvclass out"=w552:refnum<class "Universal Robot.lvclass">)  [unwired: 16 in]
          }
        }
      }
      n138 = flat-sequence {
        tunnel: w17 -> [w45]
        tunnel: w16 -> [w43]
        tunnel: w15 -> [_]
        frame #0 {
          # "cleanup events"
          n139 = Unregister For Events(event registration refnum=w45) -> (error out=w44:errorcluster)  [unwired: 1 in]
          n140 = Destroy User Event(user event=w43, error in=w44) -> ()  [unwired: 1 out]
        }
      }
      n141 = call "ProgramControlStateTracker.vi"("Universal Robot.lvclass"=w19, "Complete (F)"=w14) -> ("Universal Robot.lvclass out"=w15:refnum<class "Universal Robot.lvclass">)  [unwired: 17 in]
      n142 = Release Queue(queue=w39, error in (no error)=w40) -> (error out=w24:errorcluster)  [unwired: 1 in, 2 out]
      n143 = Generate User Event(user event=w16, event data cluster=w14) -> (user event out=w26:refnum<user-event>, error out=w25:errorcluster)  [unwired: 2 in]
      n144 = Destroy User Event(user event=w26, error in=w25) -> (error out=w13:errorcluster)
      n145 = invoke class="SubPnl" method="Remove VI"(reference=w12, error in=w13) -> (error out=w11:errorcluster)  [unwired: 1 in, 2 out]
    }
    frame Error {
    }
  }
  "error out" <- w7
  "Universal Robot.lvclass out" <- w6
  "programReturnStatus" <- w8
